vi "Initiate.vi"(8 "error in (no error)":errorcluster, 10 "Batch Group Number  (0: OFF)":i32(ring) items=["OFF", "1", "2", "3", "4", "5", "6", "7", "8", "9", "10", "11", "12", "ALL"], 11 "VISA resource name":refnum<visa-resource-name>) -> (0 "error out":errorcluster, 3 "VISA resource name out":refnum<visa-resource-name>)   [LabVIEW 2020, in "Yokogawa GX Series.lvlib"]
doc: "Initiates a waveform acquisition. After you call this VI, the instrument leaves the Idle state and waits for a trigger.\n\n<B>Note</B> This VI does not check the instrument status. Typically, you call this VI only in a sequence of calls to other low-level instrument driver VIs. The sequence performs one operation. You use the low-level VIs to optimize one or more aspects of interaction with the instrument."
uses:
  <instrlib>/Yokogawa GX Series/Yokogawa GX Series.lvlib
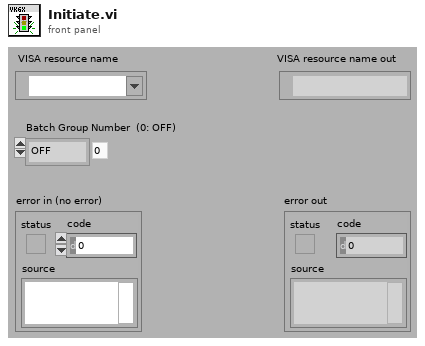
[diagram p1: front panel]
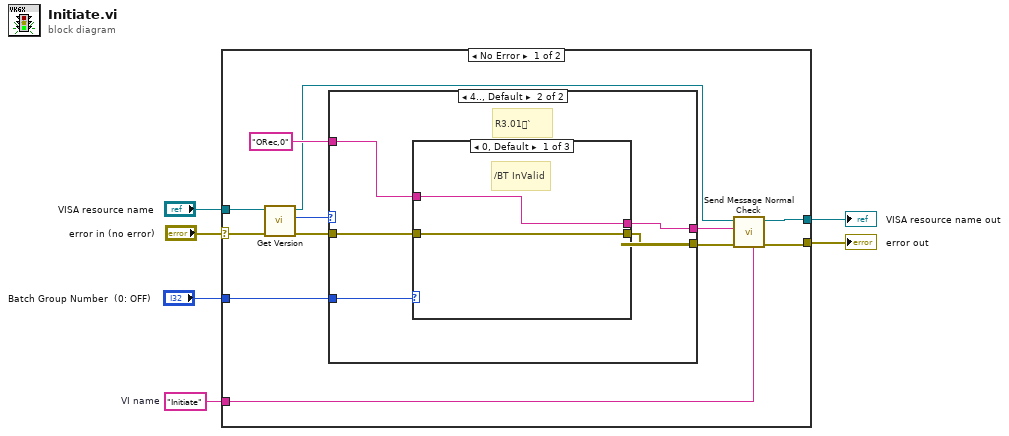
[diagram p0: block diagram]
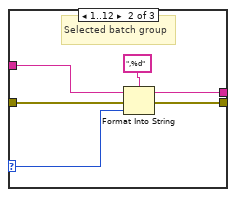
[diagram p3: hidden frame]
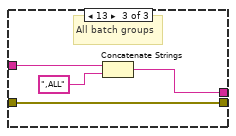
[diagram p4: hidden frame]
diagram:
  w4 = "Initiate"  # VI name
  n1 = case shown="No Error" "error in (no error)" {
    selector: "error in (no error)" -> [w14 w38]
    tunnel: "VISA resource name" -> [w15 w39]
    tunnel: [w18 w39] -> w6
    tunnel: [w17 w38] -> w5
    tunnel: w4 -> [w16 _]
    tunnel: "Batch Group Number  (0: OFF)" -> [w7 _]
    frame No Error {
      n2 = call <instrlib>:"Get Version.vi"("error in (no error)"=w14, "VISA resource name"=w15) -> ("error out"=w11:errorcluster, "Version"=w13:i32, "VISA resource name out"=w8:refnum<visa-resource-name>)  [unwired: 7 in]
      n3 = case shown="4.., Default" w13 {
        tunnel: "ORec,0" -> [w20 w25]
        tunnel: [w20 w22] -> w9
        tunnel: w11 -> [w19 w24]
        tunnel: [w19 w23] -> w10
        tunnel: w7 -> [_ w21]
        frame 0..3 {
          # "R1.03AR2.02AR2.03"
        }
        frame 4.., Default {
          # "R3.01`"
          n4 = case shown="0, Default" w21 {
            selector: w21 -> [_ w28 _]
            tunnel: w25 -> [w27 w32 w37]
            tunnel: w24 -> [w26 w31 w34]
            tunnel: [w26 w30 w34] -> w23
            tunnel: [w27 w29 w36] -> w22
            frame 0, Default {
              # "/BT InValid"
            }
            frame 1..12 {
              # "Selected batch group"
              n5 = Format Into String(format string=",%d", initial string=w32, error in=w31, w28) -> (resulting string=w29:string, error out=w30:errorcluster)
            }
            frame 13 {
              # "All batch groups"
              n6 = Concatenate Strings(w37, ",ALL") -> (w36:string)
            }
          }
        }
      }
      n7 = call <instrlib>:"Send Message Normal Check.vi"("Source (\"\")"=w16, "error in (no error)"=w10, "Send Message (\"\")"=w9, "VISA resource name"=w8) -> ("error out"=w17:errorcluster, "VISA resource name out"=w18:refnum<visa-resource-name>)  [unwired: 2 in, 4 out]
    }
    frame Error {
    }
  }
  "error out" <- w5
  "VISA resource name out" <- w6
